vi "RGB2YUV.vi"(3 "B":i32, 4 "G":i32, 5 "R":i32) -> (0 "V":dbl, 1 "U":dbl, 2 "Y":dbl)   [LabVIEW 2009]
uses:
  <vilib>/Analysis/Matrix/Numeric/Conversions/Matrix To Array - RM.vi
  <vilib>/Analysis/Matrix/Numeric/Multiply/Multiply - RM,RM.vi
  <vilib>/Analysis/Matrix/NI_Matrix.lvlib
panel:
  out "V v3":dbl
  out "Y v3":dbl
  out "U v3":dbl
  out "V v2":dbl
  out "Y v2":dbl
  out "U v2":dbl
  out "x/y":dbl[][](array[numeric])
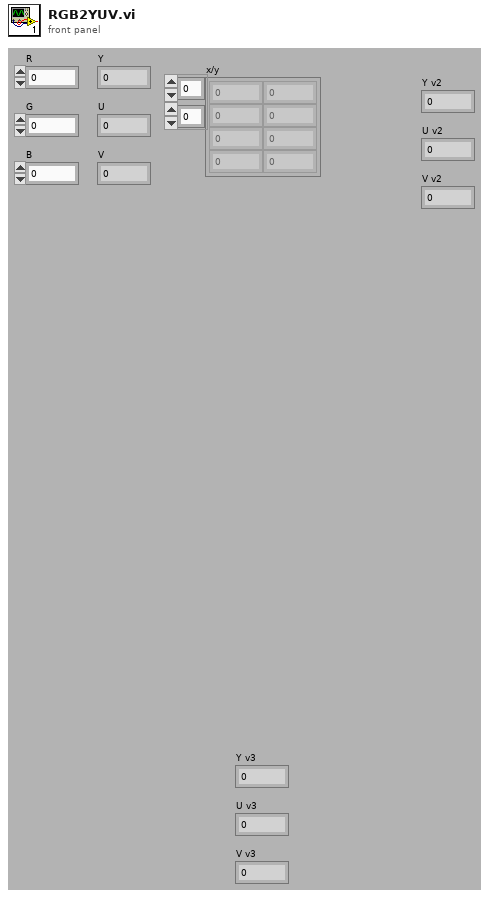
[diagram p1: front panel]
types:
  T1 = typedef "NI_Matrix.lvlib/RealMatrix.ctl" = dbl[][]
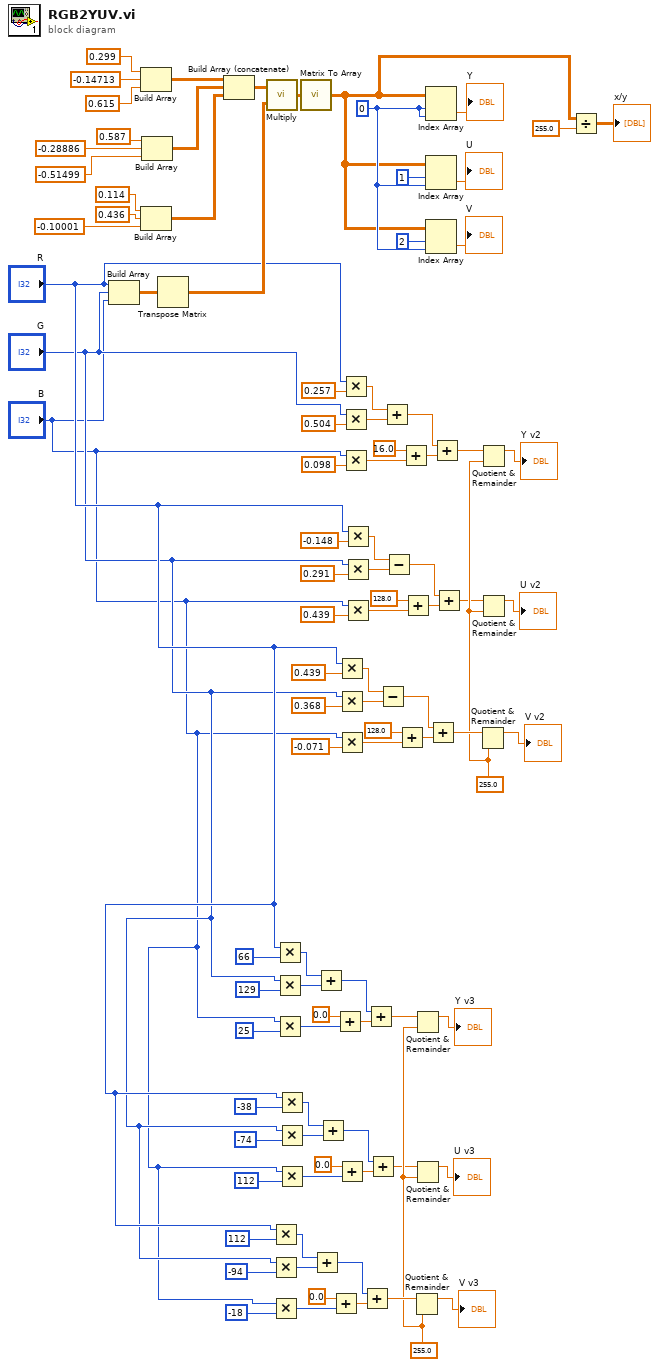
[diagram p0: block diagram]
diagram:
  w9 = 255.0 ("y")
  w43 = 255.0 ("y")
  w80 = 0 ("index (row)")
  n1 = Build Array("R", "G", "B") -> (w96:T1)
  n2 = Build Array(0.299, -0.14713, 0.615) -> (w86:T1)
  n3 = Build Array(0.114, 0.436, -0.10001) -> (w85:T1)
  n4 = Build Array(0.587, -0.28886, -0.51499) -> (w84:T1)
  n5 = Transpose Matrix(1:w96) -> (0:w82:T1)
  n6 = Build Array (concatenate)(w86, w84, w85) -> (w83:T1)
  n7 = call-poly <vilib>:"Multiply.vi"("Real Matrix B"=w82, "Real Matrix A"=w83) -> ("A * B"=w81:T1)
  n8 = Multiply(x="R", y=112) -> (x*y=w18:i32)
  n9 = Multiply(x="G", y=-94) -> (x*y=w11:i32)
  n10 = Multiply(x="B", y=-18) -> (x*y=w13:i32)
  n11 = Multiply(x="R", y=66) -> (x*y=w36:i32)
  n12 = Multiply(x="G", y=129) -> (x*y=w29:i32)
  n13 = Multiply(x="B", y=25) -> (x*y=w31:i32)
  n14 = Multiply(x="R", y=-38) -> (x*y=w27:i32)
  n15 = Multiply(x="G", y=-74) -> (x*y=w20:i32)
  n16 = Multiply(x="B", y=112) -> (x*y=w22:i32)
  n17 = call-poly <vilib>:"Matrix To Array.vi"("Real Matrix"=w81) -> ("Real 2D Array"=w73:dbl[][])
  n18 = Add(x=w18, y=w11) -> (x+y=w15:i32)
  n19 = Add(x=w36, y=w29) -> (x+y=w33:i32)
  n20 = Add(x=w27, y=w20) -> (x+y=w24:i32)
  n21 = Add(x=0.0, y=w13) -> (x+y=w14:dbl)
  n22 = Add(x=0.0, y=w31) -> (x+y=w32:dbl)
  n23 = Multiply(x="R", y=0.439) -> (x*y=w52:dbl)
  n24 = Multiply(x="G", y=0.368) -> (x*y=w45:dbl)
  n25 = Multiply(x="B", y=-0.071) -> (x*y=w47:dbl)
  n26 = Add(x=0.0, y=w22) -> (x+y=w23:dbl)
  n27 = Multiply(x="R", y=0.257) -> (x*y=w70:dbl)
  n28 = Multiply(x="G", y=0.504) -> (x*y=w63:dbl)
  n29 = Multiply(x="B", y=0.098) -> (x*y=w65:dbl)
  n30 = Multiply(x="R", y=-0.148) -> (x*y=w61:dbl)
  n31 = Multiply(x="G", y=0.291) -> (x*y=w54:dbl)
  n32 = Multiply(x="B", y=0.439) -> (x*y=w56:dbl)
  n33 = Add(x=w15, y=w14) -> (x+y=w10:dbl)
  n34 = Add(x=w33, y=w32) -> (x+y=w8:dbl)
  n35 = Add(x=w24, y=w23) -> (x+y=w7:dbl)
  n36 = Subtract(x=w52, y=w45) -> (x-y=w49:dbl)
  n37 = Add(x=w70, y=w63) -> (x+y=w67:dbl)
  n38 = Subtract(x=w61, y=w54) -> (x-y=w58:dbl)
  n39 = Add(x=128.0, y=w47) -> (x+y=w48:dbl)
  n40 = Add(x=16.0, y=w65) -> (x+y=w66:dbl)
  n41 = Add(x=128.0, y=w56) -> (x+y=w57:dbl)
  n42 = Quotient & Remainder(x=w10, y=w9) -> (x-y*floor(x/y)=→"V v3":dbl)  [unwired: 1 out]
  n43 = Quotient & Remainder(x=w8, y=w9) -> (x-y*floor(x/y)=→"Y v3":dbl)  [unwired: 1 out]
  n44 = Quotient & Remainder(x=w7, y=w9) -> (x-y*floor(x/y)=→"U v3":dbl)  [unwired: 1 out]
  n45 = Index Array(array=w73, index (row)=w80, index (col)=w80) -> (element=→"Y":dbl)
  n46 = Index Array(array=w73, index (row)=1 ("disabled index (row)"), index (col)=w80) -> (element=→"U":dbl)
  n47 = Index Array(array=w73, index (row)=2 ("disabled index (row)"), index (col)=w80) -> (element=→"V":dbl)
  n48 = Add(x=w49, y=w48) -> (x+y=w44:dbl)
  n49 = Add(x=w67, y=w66) -> (x+y=w42:dbl)
  n50 = Add(x=w58, y=w57) -> (x+y=w41:dbl)
  n51 = Quotient & Remainder(x=w44, y=w43) -> (x-y*floor(x/y)=→"V v2":dbl)  [unwired: 1 out]
  n52 = Quotient & Remainder(x=w42, y=w43) -> (x-y*floor(x/y)=→"Y v2":dbl)  [unwired: 1 out]
  n53 = Quotient & Remainder(x=w41, y=w43) -> (x-y*floor(x/y)=→"U v2":dbl)  [unwired: 1 out]
  n54 = Divide(x=w73, y=255.0) -> (x/y=→"x/y":dbl[][])
